vi "WFPropertiesNULL.vi"() -> (3 "Waveform Properties":T1={"Fs (Hz)"=20000.0, "Amplitude (V)"=5.0, "Ramp (s)"=0.0, "Duration (s)"=0.1} {"Ramp (s)" min=0.0; "Fs (Hz)" min=0.0})   [LabVIEW 2013]
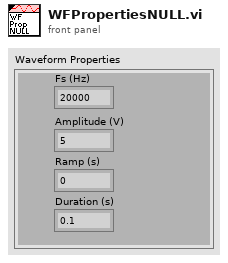
[diagram p1: front panel]
types:
  T1 = cluster{"Fs (Hz)":dbl, "Amplitude (V)":dbl, "Ramp (s)":dbl, "Duration (s)":dbl}
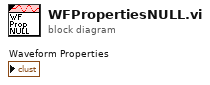
[diagram p0: block diagram]
diagram:
